vi "3.0 Timing Functional Global.vi"(2 "Grab Big Indicator":bool, 3 "Loop":T3, 4 "Read? (Write)":bool, 5 "HB In":T1) -> (0 "Timing Cluster":T2, 1 "HB Out":T1)   [LabVIEW 2010]
uses:
  4-High Neurons/4.0-Timing Badass.ctl
  3.0 List of Loops.ctl
  4-High Neurons/4.0-Timing Typedef.ctl
panel:
  out "s? t:f":T1[](array[typedef])
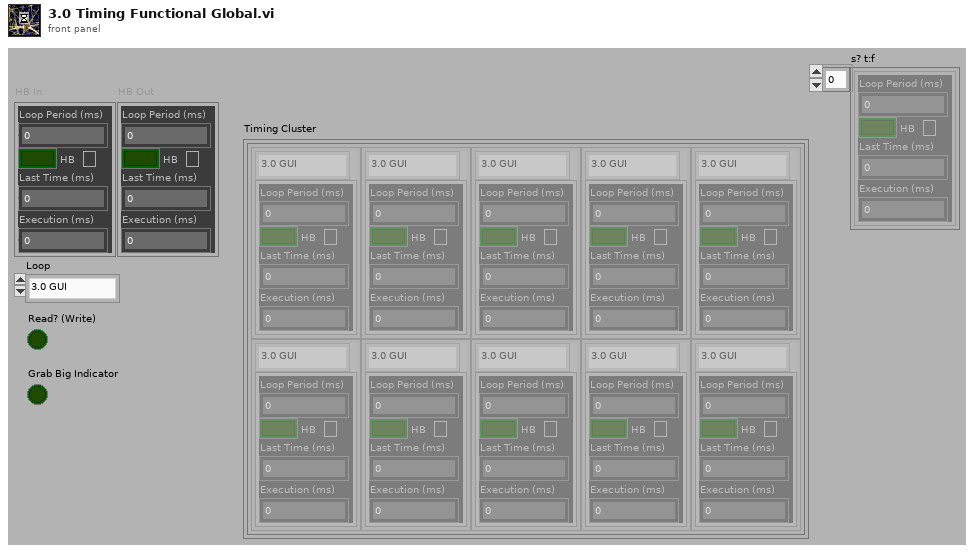
[diagram p1: front panel]
types:
  T1 = typedef "4.0-Timing Badass.ctl" = cluster{"Loop Period (ms)":u32, "HB":bool, "Last Time (ms)":u32, "Execution (ms)":u32}
  T2 = typedef "4.0-Timing Typedef.ctl" = cluster{"Array":cluster{"Loop":T3, "Super Heart Beat":T1}[][]}
  T3 = typedef "3.0 List of Loops.ctl" = enum16{"3.0 GUI", "3.1 Act", "3.1 4.7.1 Act UDP", "3.1 Joystick", "3.2 Where", "3.2 4.7.2 Where UDP", "3.3 What", "3.3 4.7.3 What UDP", "3.4 How", "3.4 4.7.4 How UDP", "3.5 Limbic", "3.6 Cerebellum"}
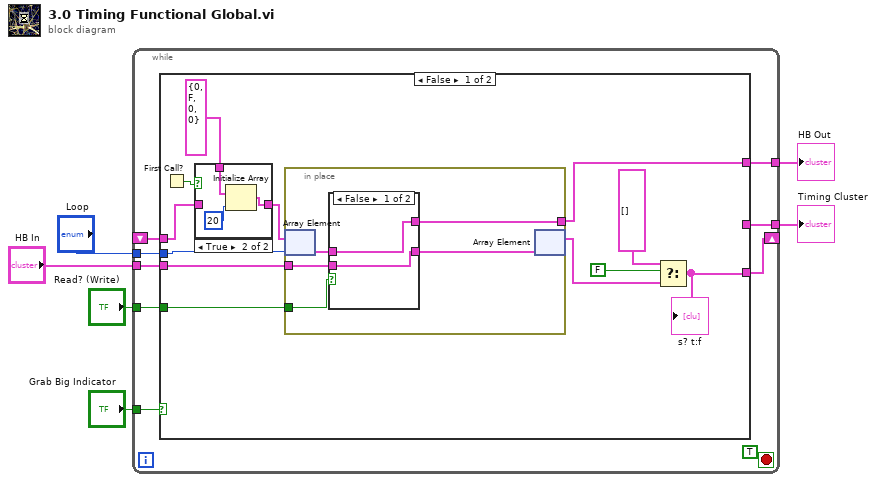
[diagram p0: block diagram]
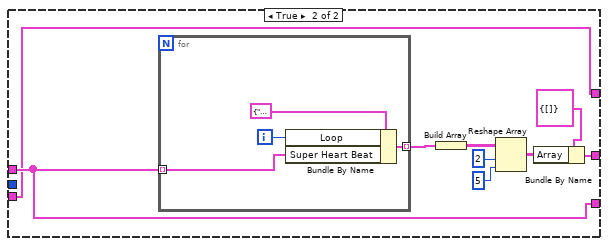
[diagram p4: hidden frame]
diagram:
  n1 = while {
    shift-right: [w10] -> _
    shift-left: _ -> [w11]
    tunnel: "Loop" -> [w15]
    tunnel: "HB In" -> [w14]
    tunnel: [w13] -> w5
    tunnel: "Read? (Write)" -> [w12]
    tunnel: "Grab Big Indicator" -> [w9]
    tunnel: [w8] -> w1
    stop <- TRUE stop-if-true
    n2 = case shown="False" w9 {
      tunnel: w15 -> [w27 _]
      tunnel: w14 -> [w26 w40]
      tunnel: [w25 w40] -> w13
      tunnel: w12 -> [w24 _]
      tunnel: w11 -> [w18 w47]
      tunnel: [w22 w47] -> w10
      tunnel: [_ w42] -> w8
      frame False {
        n3 = First Call?() -> (First Call?: T/F=w19:bool)
        n4 = case shown="True" w19 {
          tunnel: w18 -> [w28 _]
          tunnel: [w28 w29] -> w17
          tunnel: T1 {"Loop Period (ms)"=0, "HB"=FALSE, "Last Time (ms)"=0, "Execution (ms)"=0} ("HB In") -> [_ w30]
          frame False {
          }
          frame True {
            n5 = Initialize Array(w30, 20 ("dimension size")) -> (w29:T1[])
          }
        }
        n6 = in-place {
          in-place-border: w26 -> [w36]
          in-place-border: [w35] -> w25
          in-place-border: w24 -> [w34]
          n7 = in-place-array #1(w17, w27) -> (w32:T1)
          n8 = case shown="False" w34 {
            tunnel: w36 -> [w38 _]
            tunnel: [w37 w39] -> w35
            tunnel: [w38 w39] -> w33
            tunnel: w32 -> [w37 w39]
            frame False {
            }
            frame True {
            }
          }
          n9 = in-place-array #1(w33) -> (w23:T1[])  [unwired: 1 out]
        }
        n10 = Select(t=T1[] [], s=FALSE, f=w23) -> (s? t:f=w22:T1[])
        "s? t:f" <- w22
      }
      frame True {
        n11 = for {
          tunnel: w47 -> [w50] mode=indexing
          tunnel: [w49] -> w46 mode=indexing
          i -> [w51]
          n12 = Bundle By Name(cluster=cluster{"Loop":T3, "Super Heart Beat":T1} {"Loop"=enum."3.0 GUI", "Super Heart Beat"={"Loop Period (ms)"=0, "HB"=FALSE, "Last Time (ms)"=0, "Execution (ms)"=0}} ("Cluster"), "Loop"=w51, "Super Heart Beat"=w50) -> (w49:cluster{"Loop":T3, "Super Heart Beat":T1})
        }
        n13 = Build Array(w46) -> (w45:cluster{"Loop":T3, "Super Heart Beat":T1}[][])
        n14 = Reshape Array(w45, 2 ("dimension size"), 5 ("dimension size")) -> (w43:cluster{"Loop":T3, "Super Heart Beat":T1}[][])
        n15 = Bundle By Name(cluster=T2 {"Array"=[]} ("Timing Cluster"), "Array"=w43) -> (w42:T2)
      }
    }
  }
  "HB Out" <- w5
  "Timing Cluster" <- w1
